vi "Demo.vi"() -> ()   [LabVIEW 2011, in "LVH-Adept.lvlib"]
uses:
  <vilib>/LabVIEW Hacker/Adept/LVH-Adept.lvlib
  Private/DJTG/Private/Type Defs/Port Properties.ctl
  Private/DMGR/DMGR.lvlib
  Private/DJTG/DJTG.lvlib
  Private/DPCUTIL/DPCUTIL.lvlib
panel:
  out "Error Out":errorcluster
  in  "Stop Button":bool
  in  "Tab Control":T1(tab)
  in  "List Devices":bool
  in  "Dev 4":bool
  in  "Dev 3":bool
  in  "Dev 2":bool
  in  "Dev 1":bool
  in  "Dev 0":bool
  in  "Info Next":bool
  in  "Back":bool
  in  "Get JTAG Port Props":bool
  in  "Get ID Code":bool
  out "ID Codes":u32[](array[numeric]) format="%.0x"
  out "Port Properties":T2
  out "Flash Status":string
  in  "Flash Next":bool
  in  "Flash Back":bool
  in  "Flash FPGA":bool
  in  "Data":u8
  in  "Register Address":u8
  in  "RW Write":bool
  in  "RW Back":bool
  out "Data 2":u8[](array[numeric])
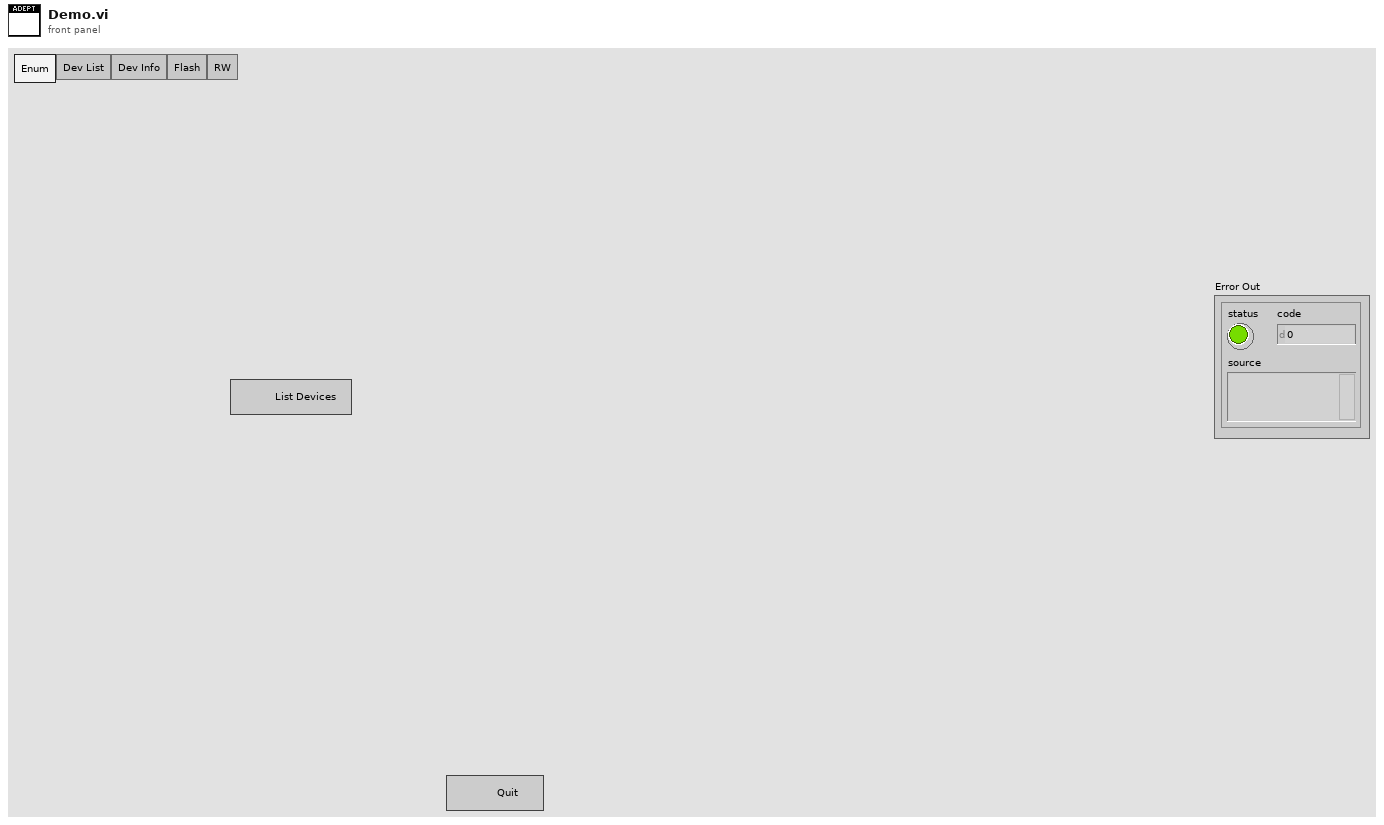
[diagram p1: front panel]
types:
  T1 = enum32{"Enum", "Dev List", "Dev Info", "Flash", "RW"}
  T2 = typedef "LVH-Adept.lvlib/DJTG.lvlib/Port Properties.ctl" = cluster{"Set Speed":bool, "Set Pin State":bool, "Trans Buffering":bool, "Wait":bool, "Delay Cnt":bool, "Ready Cnt":bool, "Escape":bool, "MScan":bool, "OScan0":bool, "OScan1":bool, "OScan2":bool, "OScan3":bool, "OScan4":bool, "OScan5":bool, "OScan6":bool, "OScan7":bool, "Check Packet":bool, "Batch":bool, "Set Aux Reset":bool}
  T3 = cluster{"Num Devices":i32, "Device Names":string[], "Devs":refnum<vi>[], "Selected Dev Num":i32, "Device Handle":u32}
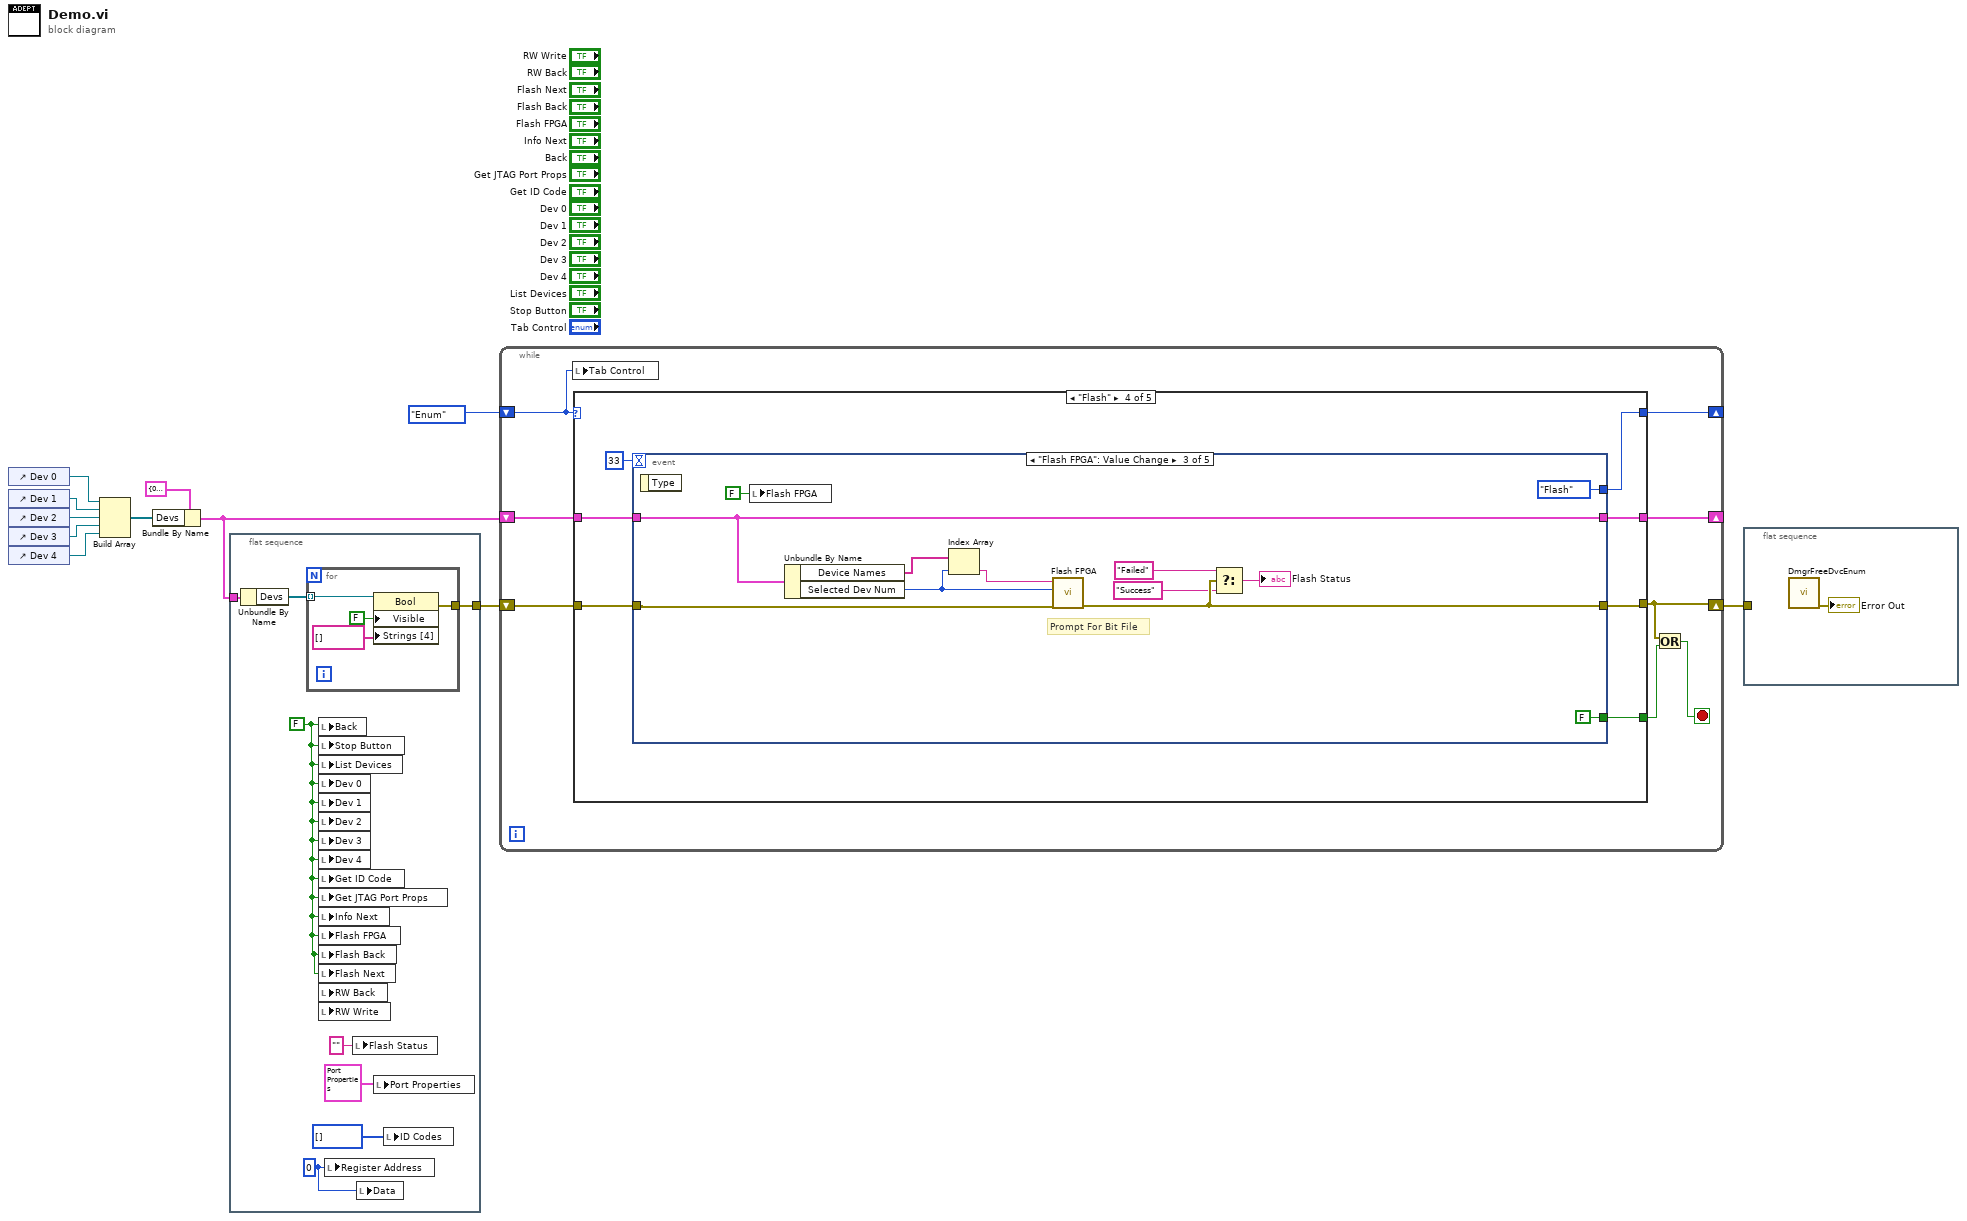
[diagram p0: block diagram]
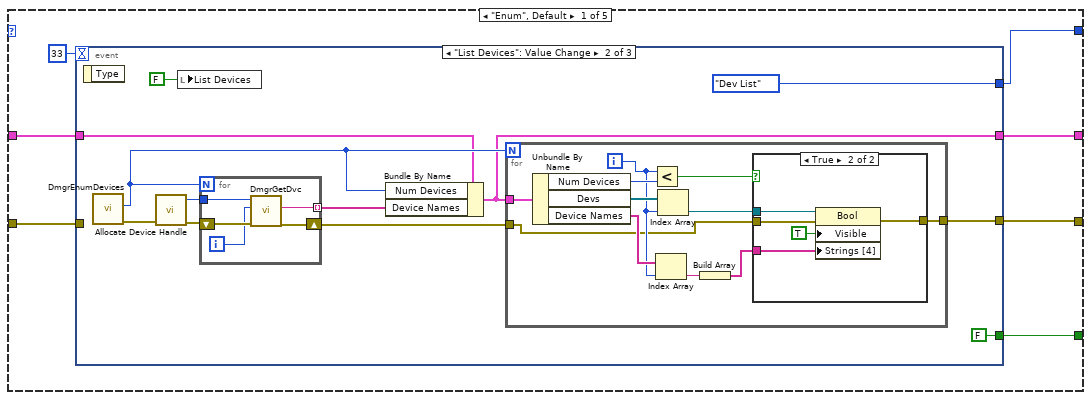
[diagram p2: hidden frame]
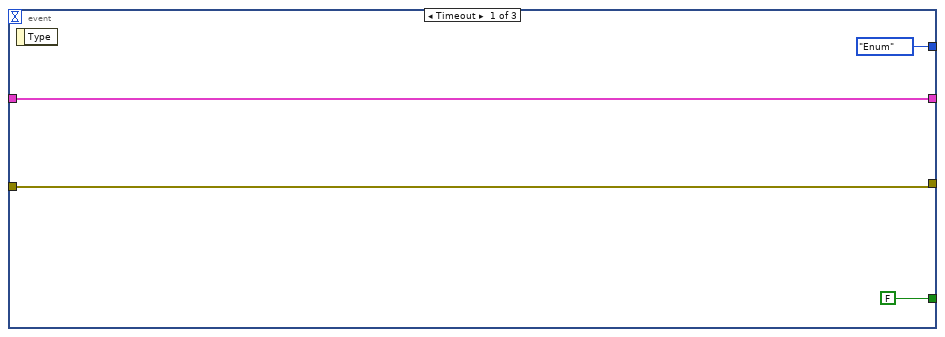
[diagram p3: hidden frame]
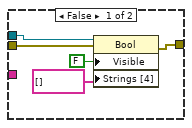
[diagram p4: hidden frame]
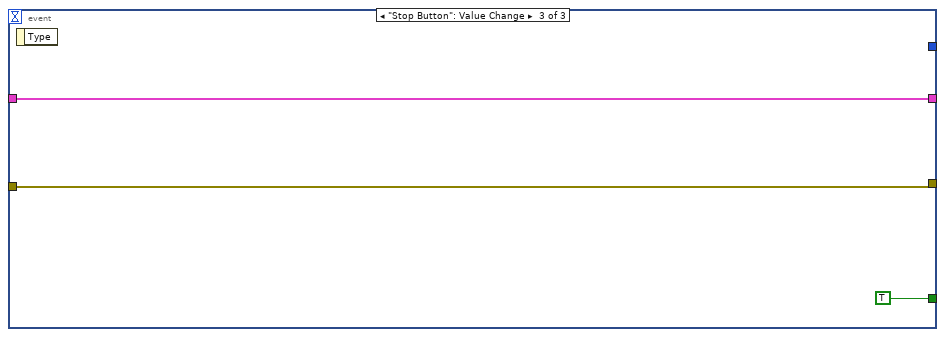
[diagram p5: hidden frame]
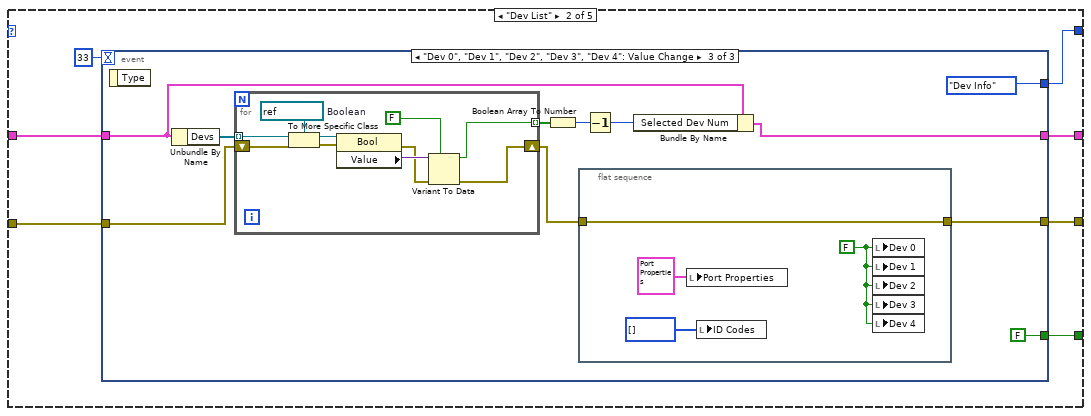
[diagram p6: hidden frame]
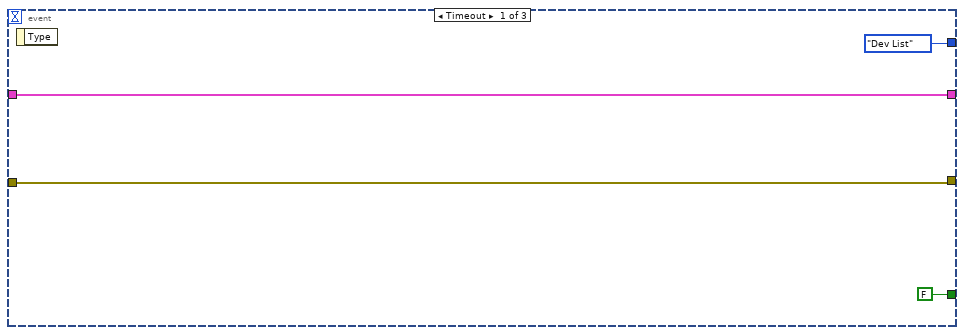
[diagram p7: hidden frame]
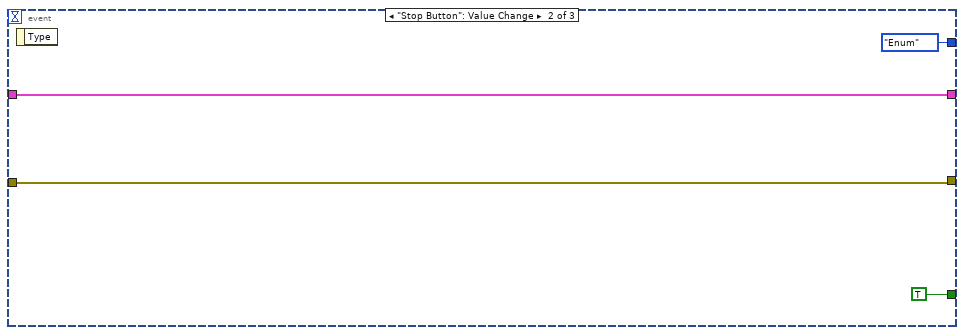
[diagram p8: hidden frame]
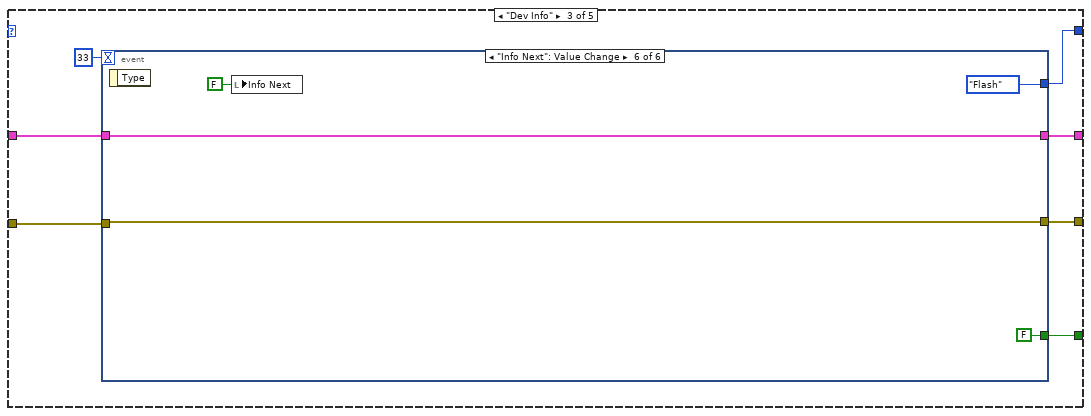
[diagram p9: hidden frame]
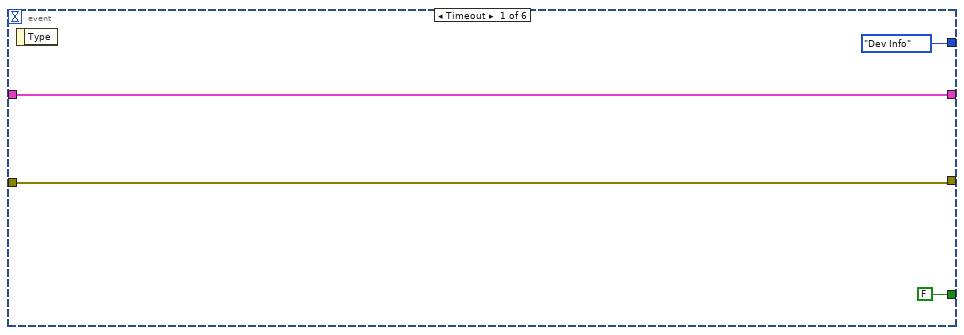
[diagram p10: hidden frame]
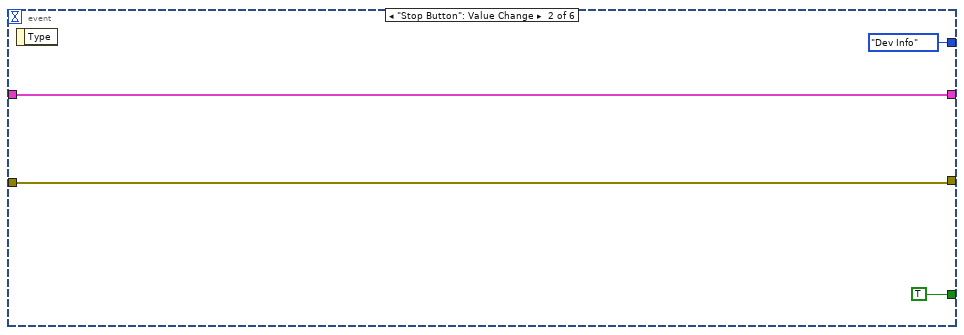
[diagram p11: hidden frame]
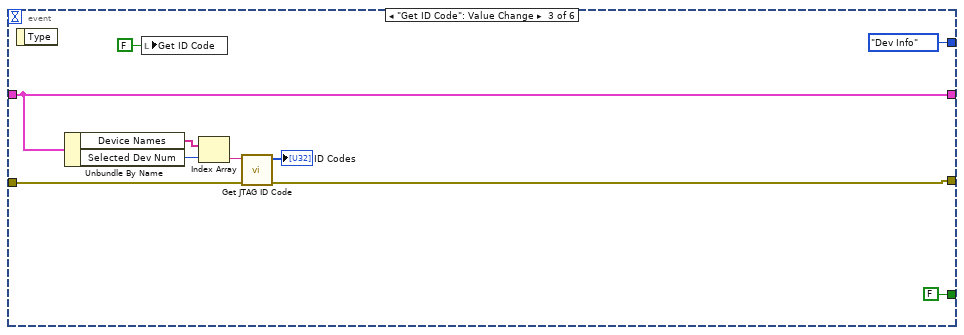
[diagram p12: hidden frame]
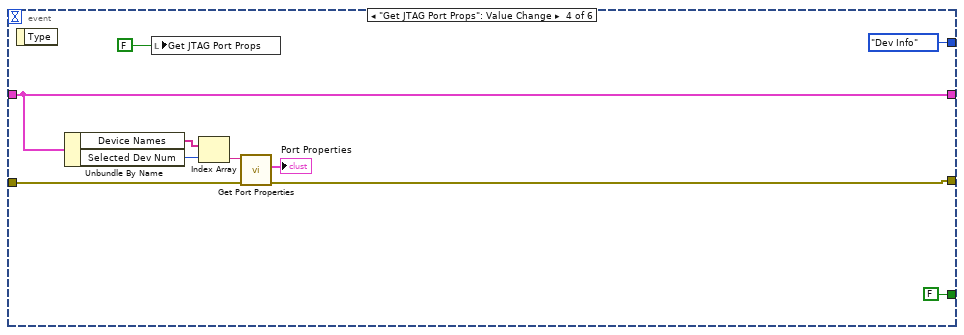
[diagram p13: hidden frame]
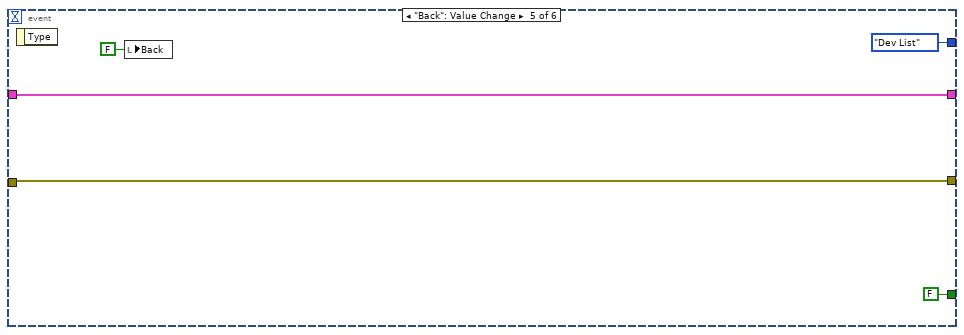
[diagram p14: hidden frame]
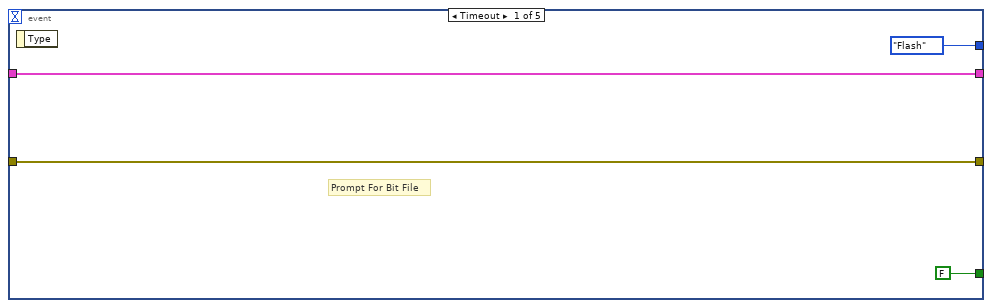
[diagram p15: hidden frame]
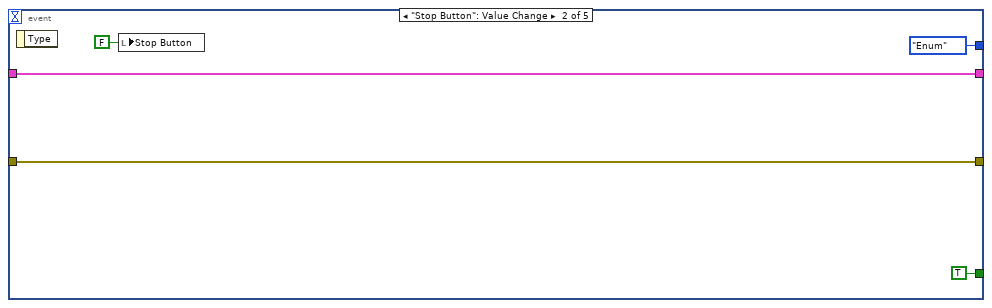
[diagram p16: hidden frame]
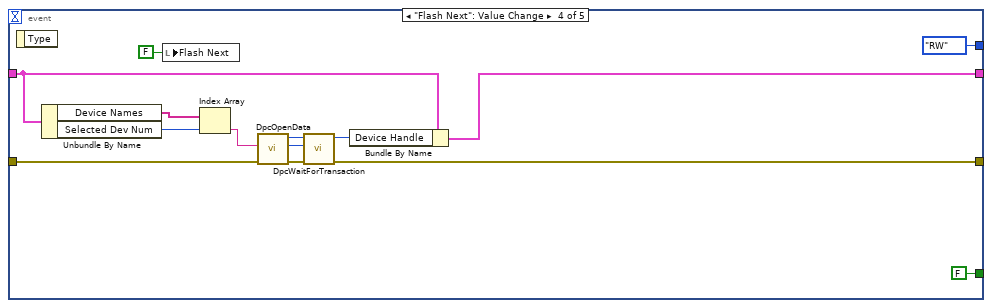
[diagram p17: hidden frame]
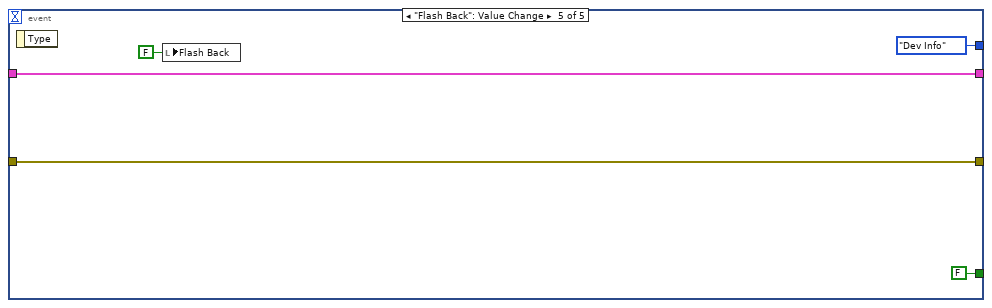
[diagram p18: hidden frame]
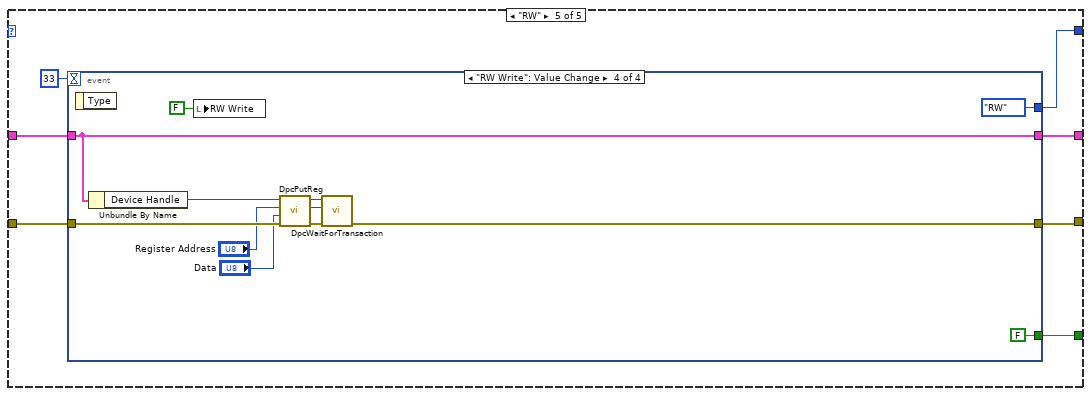
[diagram p19: hidden frame]
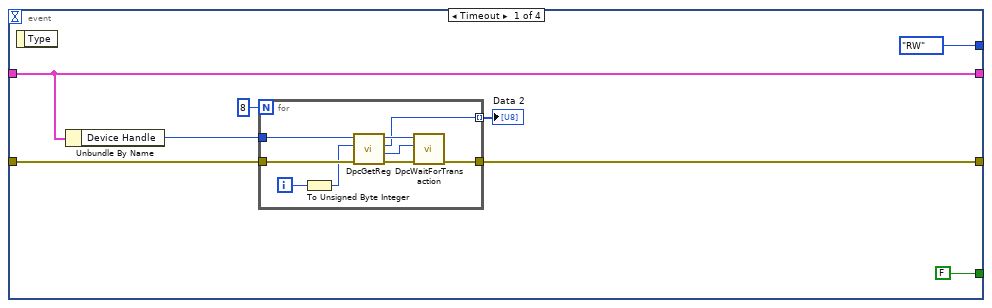
[diagram p20: hidden frame]
diagram:
  n1 = control-ref of="Dev 0"() -> (w10:refnum<vi>)
  n2 = control-ref of="Dev 1"() -> (w9:refnum<vi>)
  n3 = control-ref of="Dev 2"() -> (w8:refnum<vi>)
  n4 = control-ref of="Dev 3"() -> (w7:refnum<vi>)
  n5 = control-ref of="Dev 4"() -> (w6:refnum<vi>)
  n6 = Build Array(w10, w9, w8, w7, w6) -> (w4:refnum<vi>[])
  n7 = Bundle By Name(cluster=T3 {"Num Devices"=0, "Device Names"=[], "Devs"=[], "Selected Dev Num"=0, "Device Handle"=0}, "Devs"=w4) -> (w3:T3)
  n8 = flat-sequence {
    tunnel: [w17] -> w11
    tunnel: w3 -> [w19]
    frame #0 {
      w12 = u8 0 ("Register Address")
      w14 = FALSE ("Stop Button")
      n9 = Unbundle By Name(w19) -> ("Devs"=w18:refnum<vi>[])
      n10 = for {
        tunnel: w18 -> [w23] mode=indexing
        tunnel: [w21] -> w17
        n11 = property class="Bool"(reference=w23, "Visible"=FALSE, "Strings [4]"=string[] []) -> (error out=w21:errorcluster)  [unwired: 1 in, 1 out]
      }
      n12 = local write "Back"(w14) -> ()
      n13 = local write "Stop Button"(w14) -> ()
      n14 = local write "List Devices"(w14) -> ()
      n15 = local write "Dev 0"(w14) -> ()
      n16 = local write "Dev 1"(w14) -> ()
      n17 = local write "Dev 2"(w14) -> ()
      n18 = local write "Dev 3"(w14) -> ()
      n19 = local write "Dev 4"(w14) -> ()
      n20 = local write "Get ID Code"(w14) -> ()
      n21 = local write "Get JTAG Port Props"(w14) -> ()
      n22 = local write "Info Next"(w14) -> ()
      n23 = local write "Flash FPGA"(w14) -> ()
      n24 = local write "Flash Back"(w14) -> ()
      n25 = local write "Flash Next"(w14) -> ()
      n26 = local write "RW Back"(w14) -> ()
      n27 = local write "RW Write"(w14) -> ()
      n28 = local write "Register Address"(w12) -> ()
      n29 = local write "Flash Status"("" ("Flash Status")) -> ()
      n30 = local write "Data"(w12) -> ()
      n31 = local write "Port Properties"(T2 {"Set Speed"=FALSE, "Set Pin State"=FALSE, "Trans Buffering"=FALSE, "Wait"=FALSE, "Delay Cnt"=FALSE, "Ready Cnt"=FALSE, "Escape"=FALSE, "MScan"=FALSE, "OScan0"=FALSE, "OScan1"=FALSE, "OScan2"=FALSE, "OScan3"=FALSE, "OScan4"=FALSE, "OScan5"=FALSE, "OScan6"=FALSE, "OScan7"=FALSE, "Check Packet"=FALSE, "Batch"=FALSE, "Set Aux Reset"=FALSE} ("Port Properties")) -> ()
      n32 = local write "ID Codes"(i32[] []) -> ()
    }
  }
  n33 = while {
    shift-right: [w26] -> w1
    shift-left: w11 -> [w30]
    shift-right: [w29] -> _
    shift-left: w3 -> [w31]
    shift-right: [w28] -> _
    shift-left: T1."Enum" ("Tab Control") -> [w27]
    stop <- w24 stop-if-true
    n34 = local write "Tab Control"(w27) -> ()
    n35 = case shown="\"Flash\"" w27 {
      tunnel: w31 -> [w35 w87 w127 w171 w217]
      tunnel: w30 -> [w37 w86 w126 w175 w222]
      tunnel: [w32 w84 w124 w169 w220] -> w26
      tunnel: [w36 w88 w128 w172 w218] -> w29
      tunnel: [w34 w89 w129 w173 w219] -> w28
      tunnel: [w33 w85 w125 w170 w216] -> w25
      frame "Enum", Default {
        n36 = event shown="[1] \"List Devices\": Value Change" {
          selector: _ -> [_ _ _]
          dyn-events: _ -> [_ _ _]
          timeout: 33 -> [_ _ _]
          tunnel: [w42 w45 w83] -> w32
          tunnel: w37 -> [w42 _ w83]
          tunnel: [w41 w43 w82] -> w36
          tunnel: w35 -> [w41 w44 w82]
          tunnel: [enum32{"Enum", "Dev List"}."Enum" ("Tab Control") enum32{"Enum", "Dev List"}."Dev List" ("Tab Control") _] -> w34
          tunnel: [FALSE FALSE TRUE] -> w33
          event Timeout {
            n37 = event-data() -> ()  [unwired: 1 in, 1 out]
          }
          event "List Devices": Value Change {
            n38 = event-data() -> ()  [unwired: 1 in, 1 out]
            n39 = call "DmgrEnumDevices.vi"() -> ("Error Out"=w53:errorcluster, "Num Devices"=w47:i32)  [unwired: 10 in]
            n40 = call "Allocate Device Handle.vi"("Error In"=w53) -> ("Error Out"=w52:errorcluster, "Device Handle"=w51:u64)  [unwired: 9 in]
            n41 = local write "List Devices"(FALSE ("List Devices")) -> ()
            n42 = for {
              N: w47 -> [_]
              tunnel: w51 -> [w79]
              tunnel: [w78] -> w49 mode=indexing
              shift-right: [w77] -> w46
              shift-left: w52 -> [w80]
              i -> [w76]
              n43 = call "DmgrGetDvc.vi"("Error In"=w80, "Device Number"=w76, "Device Handle"=w79) -> ("Error Out"=w77:errorcluster, "Name"=w78:string)  [unwired: 4 in, 3 out]
            }
            n44 = Bundle By Name(cluster=w44, "Num Devices"=w47, "Device Names"=w49) -> (w43:T3)
            n45 = for {
              N: w47 -> [_]
              tunnel: [w65] -> w45
              tunnel: w43 -> [w64]
              tunnel: w46 -> [w57]
              i -> [w59]
              n46 = Unbundle By Name(w64) -> ("Num Devices"=w63:i32, "Devs"=w60:refnum<vi>[], "Device Names"=w61:string[])
              n47 = Less?(x=w59, y=w63) -> (x < y?=w62:bool)
              n48 = Index Array(array=w61, index=w59) -> (element=w56:string)
              n49 = Index Array(array=w60, index=w59) -> (element=w58:refnum<vi>)
              n50 = Build Array(w56) -> (w55:string[])
              n51 = case shown="True" w62 {
                tunnel: [w69 w71] -> w65
                tunnel: w58 -> [w67 w75]
                tunnel: w57 -> [w68 w74]
                tunnel: w55 -> [_ w72]
                frame False {
                  n52 = property class="Bool"(reference=w67, error in=w68, "Visible"=FALSE, "Strings [4]"=string[] []) -> (error out=w69:errorcluster)  [unwired: 1 out]
                }
                frame True {
                  n53 = property class="Bool"(reference=w75, error in=w74, "Visible"=TRUE, "Strings [4]"=w72) -> (error out=w71:errorcluster)  [unwired: 1 out]
                }
              }
            }
          }
          event "Stop Button": Value Change {
            n54 = event-data() -> ()  [unwired: 1 in, 1 out]
          }
        }
      }
      frame "Dev List" {
        n55 = event shown="[2] \"Dev 0\", \"Dev 1\", \"Dev 2\", \"Dev 3\", \"Dev 4\": Value Change" {
          selector: _ -> [_ _ _]
          dyn-events: _ -> [_ _ _]
          timeout: 33 -> [_ _ _]
          tunnel: [enum32{"Enum", "Dev List", "Dev Info"}."Dev List" ("Tab Control") enum32{"Enum", "Dev List", "Dev Info"}."Enum" ("Tab Control") enum32{"Enum", "Dev List", "Dev Info"}."Dev Info" ("Tab Control")] -> w89
          tunnel: [w94 w96 w102] -> w88
          tunnel: w87 -> [w94 w96 w103]
          tunnel: [w93 w97 w100] -> w84
          tunnel: w86 -> [w93 w97 w108]
          tunnel: [FALSE TRUE FALSE] -> w85
          event Timeout {
            n56 = event-data() -> ()  [unwired: 1 in, 1 out]
          }
          event "Stop Button": Value Change {
            n57 = event-data() -> ()  [unwired: 1 in, 1 out]
          }
          event "Dev 0", "Dev 1", "Dev 2", "Dev 3", "Dev 4": Value Change {
            n58 = event-data() -> ()  [unwired: 1 in, 1 out]
            n59 = Unbundle By Name(w103) -> ("Devs"=w109:refnum<vi>[])
            n60 = for {
              tunnel: w109 -> [w123] mode=indexing
              shift-right: [w115] -> w99
              shift-left: w108 -> [w121]
              tunnel: [w114] -> w107 mode=indexing
              w119 = refnum<vi> refnum  # Boolean
              n61 = To More Specific Class(target class=w119, reference=w123, error in=w121) -> (specific class reference=w122:refnum<vi>, error out=w120:errorcluster)
              n62 = property class="Bool"(reference=w122, error in=w120) -> (error out=w116:errorcluster, "Value"=w118:variant)  [unwired: 1 out]
              n63 = Variant To Data(error in=w116, type=FALSE, Variant=w118) -> (data=w114:bool, error out=w115:errorcluster)
            }
            n64 = Boolean Array To Number(Boolean array=w107) -> (number=w104:u32)
            n65 = flat-sequence {
              tunnel: [w110] -> w100
              tunnel: w99 -> [w110]
              frame #0 {
                w113 = FALSE ("Dev 0")
                n66 = local write "Port Properties"(T2 {"Set Speed"=FALSE, "Set Pin State"=FALSE, "Trans Buffering"=FALSE, "Wait"=FALSE, "Delay Cnt"=FALSE, "Ready Cnt"=FALSE, "Escape"=FALSE, "MScan"=FALSE, "OScan0"=FALSE, "OScan1"=FALSE, "OScan2"=FALSE, "OScan3"=FALSE, "OScan4"=FALSE, "OScan5"=FALSE, "OScan6"=FALSE, "OScan7"=FALSE, "Check Packet"=FALSE, "Batch"=FALSE, "Set Aux Reset"=FALSE} ("Port Properties")) -> ()
                n67 = local write "ID Codes"(i32[] []) -> ()
                n68 = local write "Dev 0"(w113) -> ()
                n69 = local write "Dev 1"(w113) -> ()
                n70 = local write "Dev 2"(w113) -> ()
                n71 = local write "Dev 3"(w113) -> ()
                n72 = local write "Dev 4"(w113) -> ()
              }
            }
            n73 = Decrement(x=w104) -> (x-1=w101:u32)
            n74 = Bundle By Name(cluster=w103, "Selected Dev Num"=w101) -> (w102:T3)
          }
        }
      }
      frame "Dev Info" {
        n75 = event shown="[5] \"Info Next\": Value Change" {
          selector: _ -> [_ _ _ _ _ _]
          dyn-events: _ -> [_ _ _ _ _ _]
          timeout: 33 -> [_ _ _ _ _ _]
          tunnel: [enum32{"Enum", "Dev List", "Dev Info"}."Dev Info" ("Tab Control") enum32{"Enum", "Dev List", "Dev Info"}."Dev Info" ("Tab Control") enum32{"Enum", "Dev List", "Dev Info"}."Dev Info" ("Tab Control") enum32{"Enum", "Dev List", "Dev Info"}."Dev Info" ("Tab Control") enum32{"Enum", "Dev List", "Dev Info"}."Dev List" ("Tab Control") T1."Flash" ("Tab Control")] -> w129
          tunnel: [w134 w136 w142 w156 w161 w164] -> w128
          tunnel: w127 -> [w134 w136 w142 w156 w161 w164]
          tunnel: [w133 w137 w143 w152 w160 w166] -> w124
          tunnel: w126 -> [w133 w137 w145 w151 w160 w166]
          tunnel: [FALSE TRUE FALSE FALSE FALSE FALSE] -> w125
          event Timeout {
            n76 = event-data() -> ()  [unwired: 1 in, 1 out]
          }
          event "Stop Button": Value Change {
            n77 = event-data() -> ()  [unwired: 1 in, 1 out]
          }
          event "Get ID Code": Value Change {
            n78 = event-data() -> ()  [unwired: 1 in, 1 out]
            n79 = Unbundle By Name(w142) -> ("Device Names"=w148:string[], "Selected Dev Num"=w147:i32)
            n80 = local write "Get ID Code"(FALSE ("Get ID Code")) -> ()
            n81 = Index Array(array=w148, index=w147) -> (element=w146:string)
            n82 = call "Get JTAG ID Code.vi"("Error In"=w145, "Device Name"=w146) -> ("Error Out"=w143:errorcluster, "ID Codes"=→"ID Codes":u32[])  [unwired: 8 in]
          }
          event "Get JTAG Port Props": Value Change {
            n83 = event-data() -> ()  [unwired: 1 in, 1 out]
            n84 = Unbundle By Name(w156) -> ("Device Names"=w158:string[], "Selected Dev Num"=w157:i32)
            n85 = local write "Get JTAG Port Props"(FALSE ("Get ID Code")) -> ()
            n86 = Index Array(array=w158, index=w157) -> (element=w150:string)
            n87 = call "Get Port Properties.vi"("Error In"=w151, "Device Name"=w150) -> ("Error Out"=w152:errorcluster, "Port Properties"=→"Port Properties":T2)  [unwired: 7 in, 1 out]
          }
          event "Back": Value Change {
            n88 = event-data() -> ()  [unwired: 1 in, 1 out]
            n89 = local write "Back"(FALSE ("Back")) -> ()
          }
          event "Info Next": Value Change {
            n90 = event-data() -> ()  [unwired: 1 in, 1 out]
            n91 = local write "Info Next"(FALSE ("Info Next")) -> ()
          }
        }
      }
      frame "Flash" {
        n92 = event shown="[2] \"Flash FPGA\": Value Change" {
          selector: _ -> [_ _ _ _ _]
          dyn-events: _ -> [_ _ _ _ _]
          timeout: 33 -> [_ _ _ _ _]
          tunnel: w175 -> [w176 w183 w185 w207 w214]
          tunnel: [w176 w183 w189 w200 w214] -> w169
          tunnel: [T1."Flash" ("Tab Control") T1."Enum" ("Tab Control") T1."Flash" ("Tab Control") T1."RW" ("Tab Control") T1."Dev Info" ("Tab Control")] -> w173
          tunnel: [w177 w182 w192 w197 w213] -> w172
          tunnel: w171 -> [w177 w182 w192 w198 w213]
          tunnel: [FALSE TRUE FALSE FALSE FALSE] -> w170
          event Timeout {
            # "Prompt For Bit File"
            n93 = event-data() -> ()  [unwired: 1 in, 1 out]
          }
          event "Stop Button": Value Change {
            n94 = event-data() -> ()  [unwired: 1 in, 1 out]
            n95 = local write "Stop Button"(FALSE ("Stop Button")) -> ()
          }
          event "Flash FPGA": Value Change {
            # "Prompt For Bit File"
            n96 = event-data() -> ()  [unwired: 1 in, 1 out]
            n97 = local write "Flash FPGA"(FALSE ("Flash FPGA")) -> ()
            n98 = Unbundle By Name(w192) -> ("Device Names"=w195:string[], "Selected Dev Num"=w194:i32)
            n99 = Index Array(array=w195, index=w194) -> (element=w193:string)
            n100 = call "Flash FPGA.vi"("Error In"=w185, "Device ID"=w194, "Device Name"=w193) -> ("Error Out"=w189:errorcluster)  [unwired: 8 in]
            n101 = Select(t="Failed", s=w189, f="Success") -> (s? t:f=→"Flash Status":string)
          }
          event "Flash Next": Value Change {
            n102 = event-data() -> ()  [unwired: 1 in, 1 out]
            n103 = Unbundle By Name(w198) -> ("Device Names"=w206:string[], "Selected Dev Num"=w205:i32)
            n104 = local write "Flash Next"(FALSE ("Flash Back")) -> ()
            n105 = Index Array(array=w206, index=w205) -> (element=w204:string)
            n106 = call "DpcOpenData.vi"("Error In"=w207, "Device Name"=w204) -> ("Error Out"=w203:errorcluster, "Task ID"=w201:u16, "Device Handle"=w202:u32)  [unwired: 7 in]
            n107 = call "DpcWaitForTransaction.vi"("Error In"=w203, "Task ID"=w201, "Device Handle"=w202) -> ("Error Out"=w200:errorcluster, "Device Handle"=w199:u32)  [unwired: 7 in]
            n108 = Bundle By Name(cluster=w198, "Device Handle"=w199) -> (w197:T3)
          }
          event "Flash Back": Value Change {
            n109 = event-data() -> ()  [unwired: 1 in, 1 out]
            n110 = local write "Flash Back"(FALSE ("Flash Back")) -> ()
          }
        }
      }
      frame "RW" {
        n111 = event shown="[3] \"RW Write\": Value Change" {
          selector: _ -> [_ _ _ _]
          dyn-events: _ -> [_ _ _ _]
          timeout: 33 -> [_ _ _ _]
          tunnel: w222 -> [w228 w243 w249 w263]
          tunnel: [w227 w240 w247 w254] -> w220
          tunnel: [T1."RW" ("Tab Control") T1."Enum" ("Tab Control") T1."Flash" ("Tab Control") T1."RW" ("Tab Control")] -> w219
          tunnel: [w226 w242 w248 w255] -> w218
          tunnel: w217 -> [w226 w242 w248 w255]
          tunnel: [FALSE TRUE FALSE FALSE] -> w216
          event Timeout {
            n112 = event-data() -> ()  [unwired: 1 in, 1 out]
            n113 = Unbundle By Name(w226) -> ("Device Handle"=w225:u32)
            n114 = for {
              N: 8 -> [_]
              tunnel: w228 -> [w239]
              tunnel: [w237] -> w227
              tunnel: w225 -> [w235]
              tunnel: [w232] -> w224 mode=indexing
              i -> [w234]
              n115 = To Unsigned Byte Integer(number=w234) -> (unsigned 8bit integer=w233:u8)
              n116 = call "DpcGetReg.vi"("Error In"=w239, "Register Address"=w233, "Device Handle"=w235) -> ("Error Out"=w238:errorcluster, "Task ID"=w231:u16, "Data"=w232:u8, "Device Handle"=w236:u32)  [unwired: 5 in]
              n117 = call "DpcWaitForTransaction.vi"("Error In"=w238, "Task ID"=w231, "Device Handle"=w236) -> ("Error Out"=w237:errorcluster)  [unwired: 7 in, 1 out]
            }
            "Data 2" <- w224
          }
          event "Stop Button": Value Change {
            n118 = event-data() -> ()  [unwired: 1 in, 1 out]
            n119 = Unbundle By Name(w242) -> ("Device Handle"=w241:u32)
            n120 = local write "Stop Button"(FALSE ("Stop Button")) -> ()
            n121 = call "DpcCloseData.vi"("Error In"=w243, "Device Handle"=w241) -> ("Error Out"=w240:errorcluster)  [unwired: 8 in, 1 out]
          }
          event "RW Back": Value Change {
            n122 = event-data() -> ()  [unwired: 1 in, 1 out]
            n123 = Unbundle By Name(w248) -> ("Device Handle"=w250:u32)
            n124 = local write "Flash Back"(FALSE ("Flash Back")) -> ()
            n125 = call "DpcCloseData.vi"("Error In"=w249, "Device Handle"=w250) -> ("Error Out"=w247:errorcluster)  [unwired: 8 in, 1 out]
          }
          event "RW Write": Value Change {
            n126 = event-data() -> ()  [unwired: 1 in, 1 out]
            n127 = Unbundle By Name(w255) -> ("Device Handle"=w262:u32)
            n128 = local write "RW Write"(FALSE ("RW Write")) -> ()
            n129 = call "DpcPutReg.vi"("Error In"=w263, "Data"="Data", "Register Address"="Register Address", "Device Handle"=w262) -> ("Error Out"=w264:errorcluster, "Task ID"=w258:u16, "Device Hanle"=w259:u32)  [unwired: 5 in]
            n130 = call "DpcWaitForTransaction.vi"("Error In"=w264, "Task ID"=w258, "Device Handle"=w259) -> ("Error Out"=w254:errorcluster)  [unwired: 7 in, 1 out]
          }
        }
      }
    }
    n131 = Or(x=w26, y=w25) -> (x .or. y?=w24:bool)
  }
  n132 = flat-sequence {
    tunnel: w1 -> [_]
    frame #0 {
      n133 = call "DmgrFreeDvcEnum.vi"() -> ("Error Out"=→"Error Out":errorcluster)  [unwired: 11 in]
    }
  }
